vi "Get_Instrument_Instance.vi"(0 "Factory in":refnum<class "InstrumentFactory.lvclass">, 5 "Factory_Data":variant, 11 "error in (no error)":errorcluster) -> (4 "Factory out":refnum<class "InstrumentFactory.lvclass">, 6 "Instruments":refnum<class "Abstract_Instrument.lvclass">[](array[class]), 15 "error out":errorcluster)   [LabVIEW 2020, in "InstrumentFactory.lvlib" / "InstrumentFactory.lvclass"]
uses:
  InstrumentFactory.lvclass
  Abstract_Instrument/Base/Abstract_Instrument.lvclass
  InstrumentFactory.lvclass/InstrumentFactory.ctl
  <vilib>/MeasurementLink/MeasurementLink Session Management V1/Session Reservation/Session Reservation.lvclass/Session Reservation.ctl
  <vilib>/MeasurementLink/MeasurementLink Session Management V1/Session Reservation/Get Session Info - NSess .vi
  <vilib>/MeasurementLink/MeasurementLink Session Management V1/Session Reservation/Merge Invalid DVR Error.vi
  <vilib>/MeasurementLink/MeasurementLink Session Management V1/Session Reservation/Is DVR Valid.vi
  <vilib>/MeasurementLink/MeasurementLink Measurement Server/Helpers/Error Strings Global Internal.vi
  <vilib>/Utility/error.llb/Error Cluster From Error Code.vi
  <vilib>/MeasurementLink/MeasurementLink Session Management V1/Session Reservation/Session Reservation.lvclass
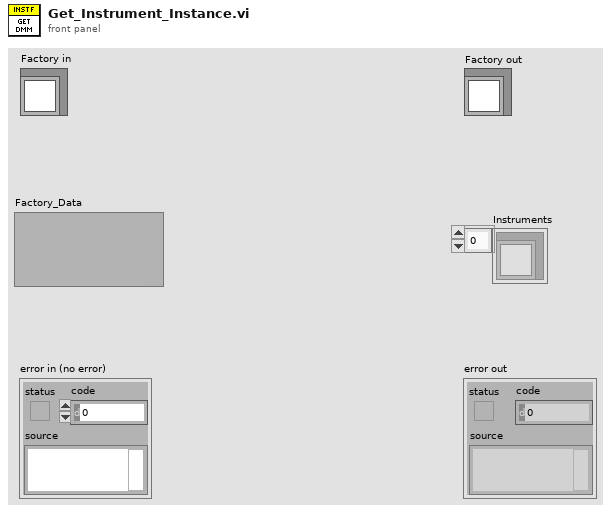
[diagram p1: front panel]
types:
  T1 = typedef "InstrumentFactory.lvlib/InstrumentFactory.lvclass/Factory_Data.ctl" = cluster{"session reservation in":refnum<class "Session Reservation.lvclass">}
  T2 = typedef "MeasurementLink Session Management Client.lvlib/ni_measurementlink_sessionmanagement_v1_SessionInformation.ctl" = cluster{"session":T3, "resource_name":string, "channel_list":string, "instrument_type_id":string, "session_exists":bool, "channel_mappings":T4[]}
  T3 = typedef "MeasurementLink Session Management Client.lvlib/nidevice_grpc_Session.ctl" = cluster{"name":string}
  T4 = typedef "MeasurementLink Session Management Client.lvlib/ni_measurementlink_sessionmanagement_v1_ChannelMapping.ctl" = cluster{"pin_or_relay_name":string, "site":i32, "channel":string, "multiplexer_resource_name":string, "multiplexer_route":string}
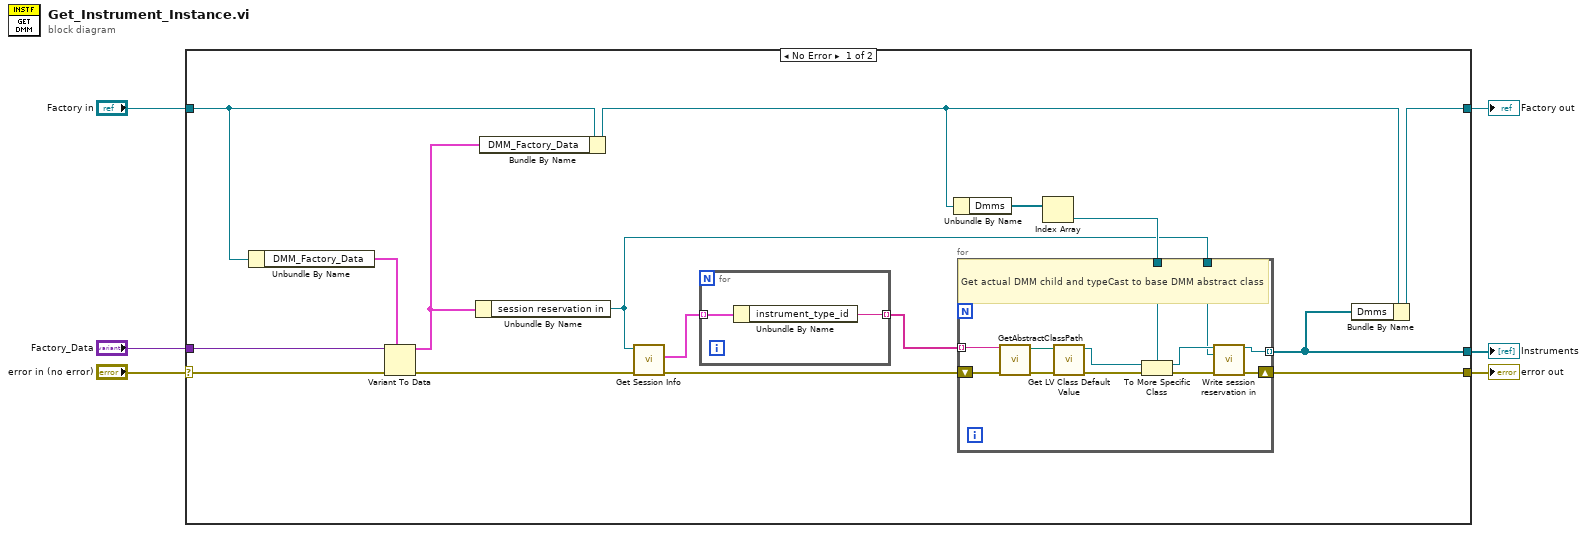
[diagram p0: block diagram]
diagram:
  n1 = case shown="No Error" "error in (no error)" {
    selector: "error in (no error)" -> [w22 w38]
    tunnel: [w19 w38] -> w5
    tunnel: [w12 w37] -> w3
    tunnel: "Factory in" -> [w15 w37]
    tunnel: "Factory_Data" -> [w17 _]
    tunnel: [w9 _] -> w1
    frame No Error {
      n2 = Unbundle By Name(w15) -> ("DMM_Factory_Data"=w16:T1)
      n3 = Variant To Data(error in=w22, type=w16, Variant=w17) -> (data=w10:T1, error out=w18:errorcluster)
      n4 = Unbundle By Name(w10) -> ("session reservation in"=w7:refnum<class "Session Reservation.lvclass">)
      n5 = Bundle By Name(cluster=w15, "DMM_Factory_Data"=w10) -> (w11:refnum<class "InstrumentFactory.lvclass">)
      n6 = call-poly <vilib>:"Get Session Info.vi"("error in"=w18, "session reservation in"=w7) -> ("error out"=w21:errorcluster, "sessions info"=w8:T2[])  [unwired: 7 in, 1 out]
      n7 = for {
        tunnel: [w24] -> w20 mode=indexing
        tunnel: w8 -> [w23] mode=indexing
        n8 = Unbundle By Name(w23) -> ("instrument_type_id"=w24:string)
      }
      n9 = Unbundle By Name(w11) -> ("Dmms"=w14:refnum<class "Abstract_Instrument.lvclass">[])
      n10 = Index Array(array=w14) -> (element=w13:refnum<class "Abstract_Instrument.lvclass">)  [unwired: 1 in]
      n11 = for {
        tunnel: w20 -> [w34] mode=indexing
        shift-right: [w28] -> w19
        shift-left: w21 -> [w36]
        tunnel: w13 -> [w29]
        tunnel: [w26] -> w9 mode=indexing
        tunnel: w7 -> [w25]
        # "Get actual DMM child and typeCast to base DMM abstract class"
        n12 = call "GetAbstractClassPath.vi"("instrument_type_id"=w34, "error in (no error)"=w36) -> ("appended path"=w32:path, "error out"=w35:errorcluster)  [unwired: 12 in]
        n13 = call <vilib>:"Get LV Class Default Value.vi"("error in (no error)"=w35, "class path"=w32) -> ("error out"=w33:errorcluster, "object"=w30:refnum<class>)  [unwired: 8 in]
        n14 = To More Specific Class(target class=w29, reference=w30, error in=w33) -> (specific class reference=w27:refnum<class "Abstract_Instrument.lvclass">, error out=w31:errorcluster)
        n15 = call-dynamic "Write session reservation in.vi"("AbstractDMM in"=w27, "MeasurementLink Session Management V1.lvlib:Session Reservation.lvclass"=w25, "error in (no error)"=w31) -> ("AbstractDMM out"=w26:refnum<class "Abstract_Instrument.lvclass">, "error out"=w28:errorcluster)  [unwired: 11 in]
      }
      n16 = Bundle By Name(cluster=w11, "Dmms"=w9) -> (w12:refnum<class "InstrumentFactory.lvclass">)
    }
    frame Error {
    }
  }
  "error out" <- w5
  "Factory out" <- w3
  "Instruments" <- w1
